vi "SwerveDriveKinematicsConstraint_New.vi"(9 "SwerveKinematics":T1 {"PrevCoR"."Y" format="%14.3f"; "PrevCoR"."X" format="%14.3f"; "Modules"."Y" format="%14.3f"; "Modules"."X" format="%14.3f"}, 11 "Max Speed (M/S)":dbl format="%20.4f") -> (3 "SWERVE_DRIVE_KINE_CONSTRAINT":T4 {"SwerveKinematics"."PrevCoR"."Y" format="%14.3f"; "SwerveKinematics"."PrevCoR"."X" format="%14.3f"; "SwerveKinematics"."Modules"."Y" format="%14.3f"; "SwerveKinematics"."Modules"."X" format="%14.3f"; "Max Speed (M/S)" format="%20.4f"})   [LabVIEW 2019, in "Trajectory_Library.lvlib"]
doc: "Constructs a swerve drive dynamics constraint.\n\nParameters:\n - maxVelocity - Maximum allowed velocity.\n - SwerveDriveKinematics - Data structure\n\nReturns\n - SwerveDriveKinematicsConstraint - Constraint data structure"
uses:
  Trajectory_Library.lvlib
  TRAJ_CONSTRAINT_SWERVE_DRIVE_KINEMATICS.ctl
  SWERVE_DRIVE_KINEMATICS.ctl
  <vilib>/Analysis/Matrix/Datatypes/RealMatrix.ctl
  TRANSLATION2D.ctl
  <vilib>/Analysis/Matrix/NI_Matrix.lvlib
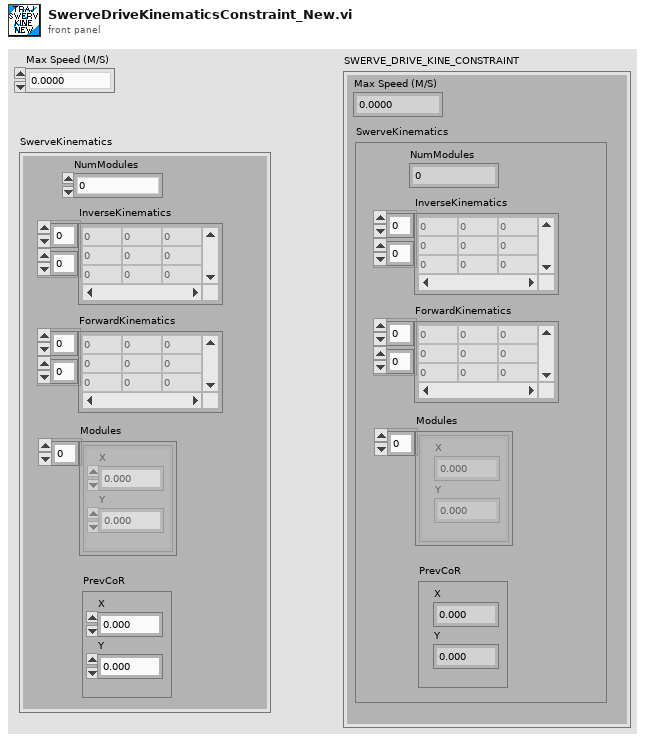
[diagram p1: front panel]
types:
  T1 = typedef "Trajectory_Library.lvlib/SWERVE_DRIVE_KINEMATICS.ctl" = cluster{"NumModules":i32, "InverseKinematics":T2, "ForwardKinematics":T2, "Modules":T3[], "PrevCoR":T3}
  T2 = typedef "NI_Matrix.lvlib/RealMatrix.ctl" = dbl[][]
  T3 = typedef "Trajectory_Library.lvlib/TRANSLATION2D.ctl" = cluster{"X":dbl, "Y":dbl}
  T4 = typedef "Trajectory_Library.lvlib/TRAJ_CONSTRAINT_SWERVE_DRIVE_KINEMATICS.ctl" = cluster{"Max Speed (M/S)":dbl, "SwerveKinematics":T1}
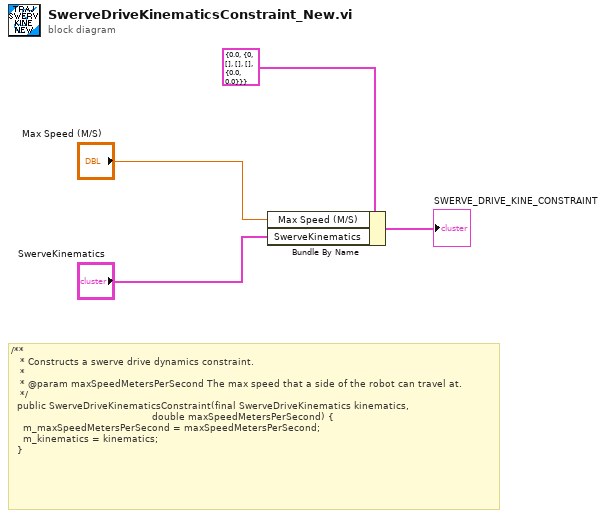
[diagram p0: block diagram]
diagram:
  # "/**\n   * Constructs a swerve drive dynamics constraint.\n   *\n   * @param maxSpeedMetersPerSecond The max speed that a side of the robot can travel at.\n   */\n  public SwerveDriveKinematicsConstraint(final SwerveDriveKinematics kinematics,\n                                               double maxSpeedMetersPerSecond) {\n    m_maxSpeedMetersPerSecond = maxSpeedMetersPerSecond;\n    m_kinematics = kinematics;\n  }"
  n1 = Bundle By Name(cluster=T4 {"Max Speed (M/S)"=0.0, "SwerveKinematics"={"NumModules"=0, "InverseKinematics"=[], "ForwardKinematics"=[], "Modules"=[], "PrevCoR"={"X"=0.0, "Y"=0.0}}} ("SWERVE_DRIVE_KINE_CONSTRAINT"), "Max Speed (M/S)"="Max Speed (M/S)", "SwerveKinematics"="SwerveKinematics") -> (→"SWERVE_DRIVE_KINE_CONSTRAINT":T4)
